vi "Init(Camera).vi"(8 "error in (no error)":errorcluster, 10 "Camera_Settings_Ref":refnum<vi>, 11 "Session in":T1) -> (0 "error out":errorcluster, 3 "Session out":T1)   [LabVIEW 2020]
uses:
  <vilib>/userDefined/High Color/IMAQdx.ctl
  Controls/Camera_Settings.ctl
  <resource>/objmgr/imaqdx.rc
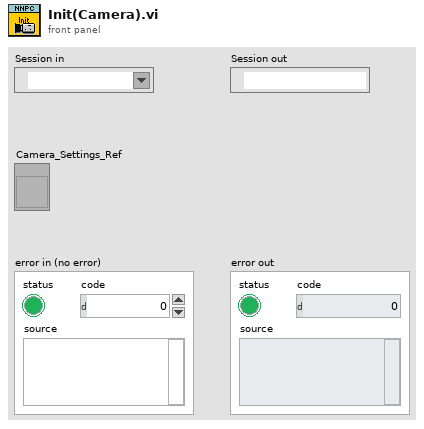
[diagram p1: front panel]
types:
  T1 = typedef "IMAQdx.ctl" = refnum<k21>
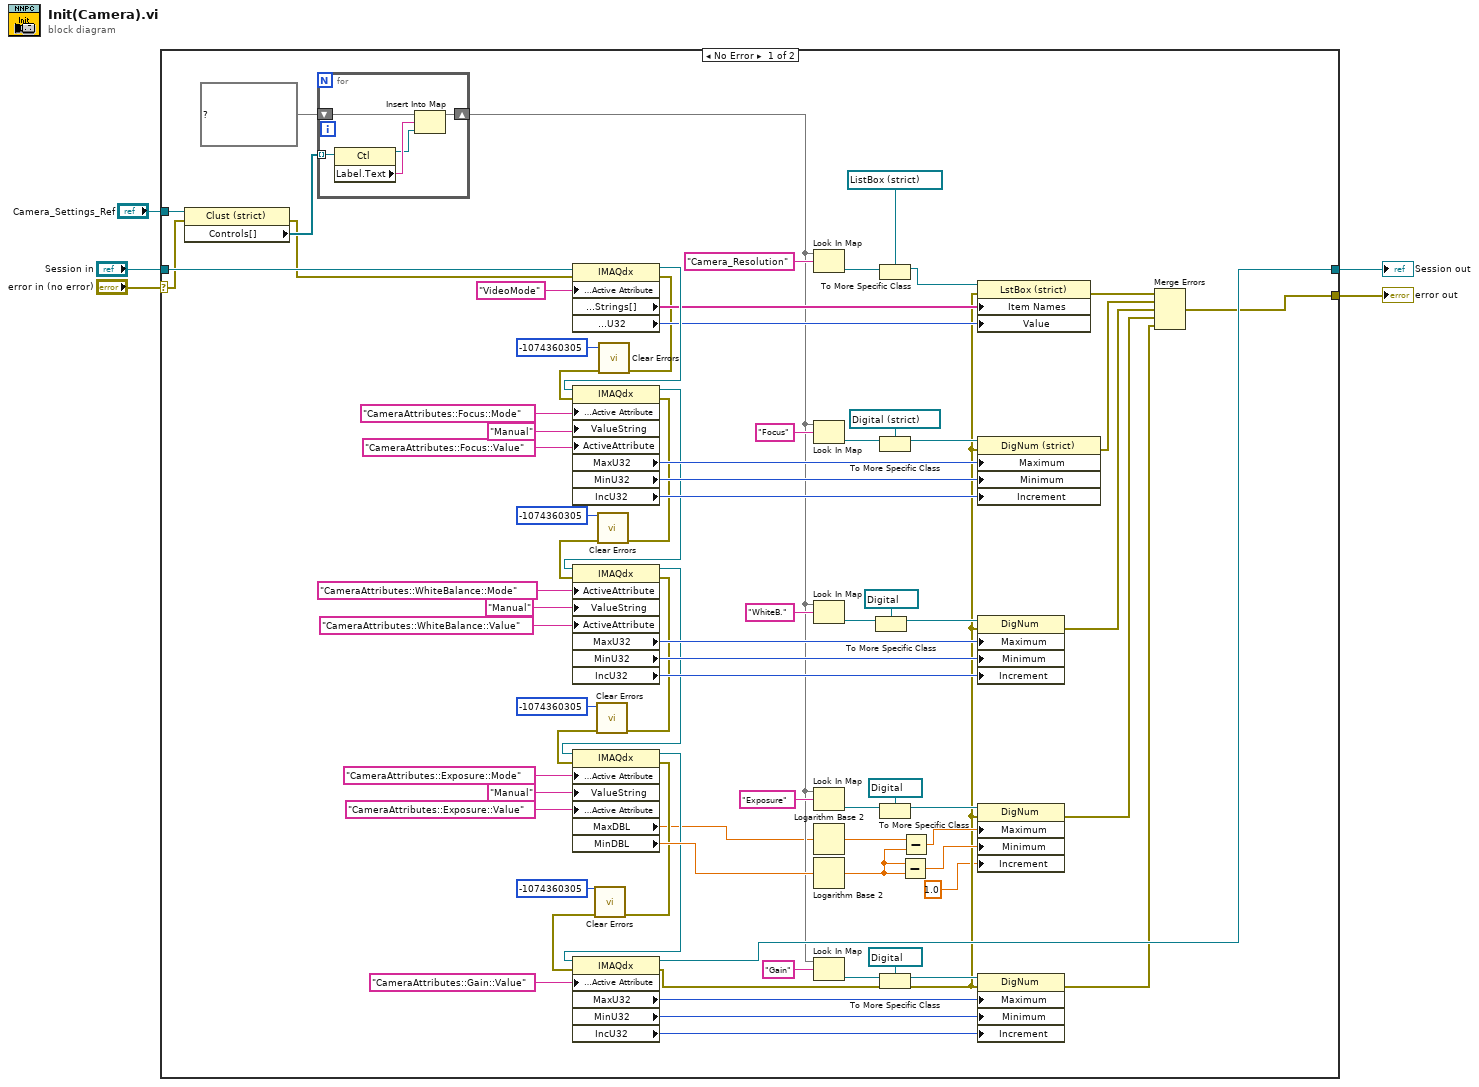
[diagram p0: block diagram]
diagram:
  n1 = case shown="No Error" "error in (no error)" {
    selector: "error in (no error)" -> [w41 w92]
    tunnel: [w74 w91] -> w5
    tunnel: [w16 w92] -> w4
    tunnel: "Camera_Settings_Ref" -> [w65 _]
    tunnel: "Session in" -> [w42 w91]
    frame No Error {
      n2 = property class="Clust (strict)"(reference=w65, error in=w41) -> (error out=w40:errorcluster, "Controls[]"=w64:refnum<vi>[])  [unwired: 1 out]
      n3 = for {
        tunnel: w64 -> [w90] mode=indexing
        shift-right: [w86] -> w28
        shift-left: map{string, refnum<vi>} {} ("map") -> [w89]
        n4 = property class="Ctl"(reference=w90) -> (reference out=w87:refnum<vi>, "Label.Text"=w88:string)  [unwired: 1 in, 1 out]
        n5 = Insert Into Map(map in=w89, key=w88, value=w87) -> (map out=w86:map{string, refnum<vi>})  [unwired: 2 out]
      }
      n6 = property class="IMAQdx"(reference=w42, error in=w40, "Camera Attributes:Active Attribute"="VideoMode" ("ActiveAttribute")) -> (reference out=w69:T1, error out=w26:errorcluster, "Camera Attributes:Enum:Strings[]"=w67:string[], "Camera Attributes:Value:U32"=w68:u32)
      n7 = call <vilib>:"Clear Errors.vi"("error in (no error)"=w26, "specific error code to clear (0: all)"=-1074360305) -> ("error out"=w15:errorcluster)  [unwired: 4 in, 1 out]
      n8 = property class="IMAQdx"(reference=w69, error in=w15, "Camera Attributes:Active Attribute"="CameraAttributes::Focus::Mode" ("ActiveAttribute"), "ValueString"="Manual", "ActiveAttribute"="CameraAttributes::Focus::Value") -> (reference out=w48:T1, error out=w27:errorcluster, "MaxU32"=w83:u32, "MinU32"=w84:u32, "IncU32"=w85:u32)
      n9 = call <vilib>:"Clear Errors.vi"("error in (no error)"=w27, "specific error code to clear (0: all)"=-1074360305) -> ("error out"=w14:errorcluster)  [unwired: 4 in, 1 out]
      n10 = property class="IMAQdx"(reference=w48, error in=w14, "ActiveAttribute"="CameraAttributes::WhiteBalance::Mode", "ValueString"="Manual", "ActiveAttribute"="CameraAttributes::WhiteBalance::Value") -> (reference out=w47:T1, error out=w25:errorcluster, "MaxU32"=w52:u32, "MinU32"=w53:u32, "IncU32"=w54:u32)
      n11 = call <vilib>:"Clear Errors.vi"("error in (no error)"=w25, "specific error code to clear (0: all)"=-1074360305) -> ("error out"=w13:errorcluster)  [unwired: 4 in, 1 out]
      n12 = property class="IMAQdx"(reference=w47, error in=w13, "Camera Attributes:Active Attribute"="CameraAttributes::Exposure::Mode" ("ActiveAttribute"), "ValueString"="Manual", "Camera Attributes:Active Attribute"="CameraAttributes::Exposure::Value" ("ActiveAttribute")) -> (reference out=w73:T1, error out=w24:errorcluster, "MaxDBL"=w23:dbl, "MinDBL"=w79:dbl)
      n13 = call <vilib>:"Clear Errors.vi"("error in (no error)"=w24, "specific error code to clear (0: all)"=-1074360305) -> ("error out"=w12:errorcluster)  [unwired: 4 in, 1 out]
      n14 = property class="IMAQdx"(reference=w73, error in=w12, "Camera Attributes:Active Attribute"="CameraAttributes::Gain::Value" ("ActiveAttribute")) -> (reference out=w74:T1, error out=w20:errorcluster, "MaxU32"=w72:u32, "MinU32"=w71:u32, "IncU32"=w6:u32)
      n15 = Look In Map(map=w28, key="Camera_Resolution") -> (value=w37:refnum<vi>)  [unwired: 1 in, 1 out]
      n16 = Look In Map(map=w28, key="Focus") -> (value=w32:refnum<vi>)  [unwired: 1 in, 1 out]
      n17 = Look In Map(map=w28, key="WhiteB.") -> (value=w31:refnum<vi>)  [unwired: 1 in, 1 out]
      n18 = Look In Map(map=w28, key="Exposure") -> (value=w30:refnum<vi>)  [unwired: 1 in, 1 out]
      n19 = Logarithm Base 2(1:w23) -> (0:w77:dbl)
      n20 = Logarithm Base 2(1:w79) -> (0:w78:dbl)
      n21 = Look In Map(map=w28, key="Gain") -> (value=w29:refnum<vi>)  [unwired: 1 in, 1 out]
      n22 = To More Specific Class(target class=refnum<vi> refnum ("DigNum Refnum"), reference=w31) -> (specific class reference=w58:refnum<vi>)  [unwired: 1 in, 1 out]
      n23 = To More Specific Class(target class=refnum<vi> refnum ("ListBox in"), reference=w37) -> (specific class reference=w56:refnum<vi>)  [unwired: 1 in, 1 out]
      n24 = To More Specific Class(target class=refnum<vi> refnum ("DigNum Refnum 5"), reference=w32) -> (specific class reference=w55:refnum<vi>)  [unwired: 1 in, 1 out]
      n25 = To More Specific Class(target class=refnum<vi> refnum ("DigNum Refnum"), reference=w30) -> (specific class reference=w60:refnum<vi>)  [unwired: 1 in, 1 out]
      n26 = To More Specific Class(target class=refnum<vi> refnum ("DigNum Refnum"), reference=w29) -> (specific class reference=w59:refnum<vi>)  [unwired: 1 in, 1 out]
      n27 = Subtract(x=w78, y=w78) -> (x-y=w81:dbl)
      n28 = Subtract(x=w77, y=w78) -> (x-y=w80:dbl)
      n29 = property on="Property Node" class="LstBox (strict)"(reference=w56, error in=w20, "Item Names"=w67, "Value"=w68) -> (error out=w22:errorcluster)  [unwired: 1 out]
      n30 = property on="Property Node" class="DigNum (strict)"(reference=w55, error in=w20, "Maximum"=w83, "Minimum"=w84, "Increment"=w85) -> (error out=w21:errorcluster)  [unwired: 1 out]
      n31 = property on="Property Node" class="DigNum"(reference=w58, error in=w20, "Maximum"=w52, "Minimum"=w53, "Increment"=w54) -> (error out=w19:errorcluster)  [unwired: 1 out]
      n32 = property on="Property Node" class="DigNum"(reference=w60, error in=w20, "Maximum"=w80, "Minimum"=w81, "Increment"=1.0 ("Data Entry Limits:Increment")) -> (error out=w18:errorcluster)  [unwired: 1 out]
      n33 = property on="Property Node" class="DigNum"(reference=w59, error in=w20, "Maximum"=w72, "Minimum"=w71, "Increment"=w6) -> (error out=w17:errorcluster)  [unwired: 1 out]
      n34 = Merge Errors(w22, w21, w19, w18, w17) -> (w16:errorcluster)
    }
    frame Error {
    }
  }
  "Session out" <- w5
  "error out" <- w4
